vi "ejer9.vi"() -> ()   [LabVIEW 2014]
panel:
  out "Circuito resonante":bool
  in  "VRMS":dbl
  in  "Fase de V":dbl
  in  "Frec del V":dbl
  in  "Resistencia.":dbl
  in  "Capacitancia":dbl
  in  "Inductancia":dbl
  out "Voltaje Fuente":dynamicdata(graph) caption="Sine"
  out "Corriente Circuito":dynamicdata(graph) caption="Sine"
  out "Voltaje  Inductor":dynamicdata(graph) caption="Sine"
  out "Voltaje Capacitor":dynamicdata(graph) caption="Sine"
  out "Voltaje  Resistencia":dynamicdata(graph) caption="Sine"
  out "Impedancia":cdb
  out "Frec de Resonancia.":dbl
  out "IRMS":dbl
  out "Fase de I":dbl
  out "V Inductor":cdb
  out "V Capacitor":cdb
  out "V Resistencia":cdb
  in  "stop":bool
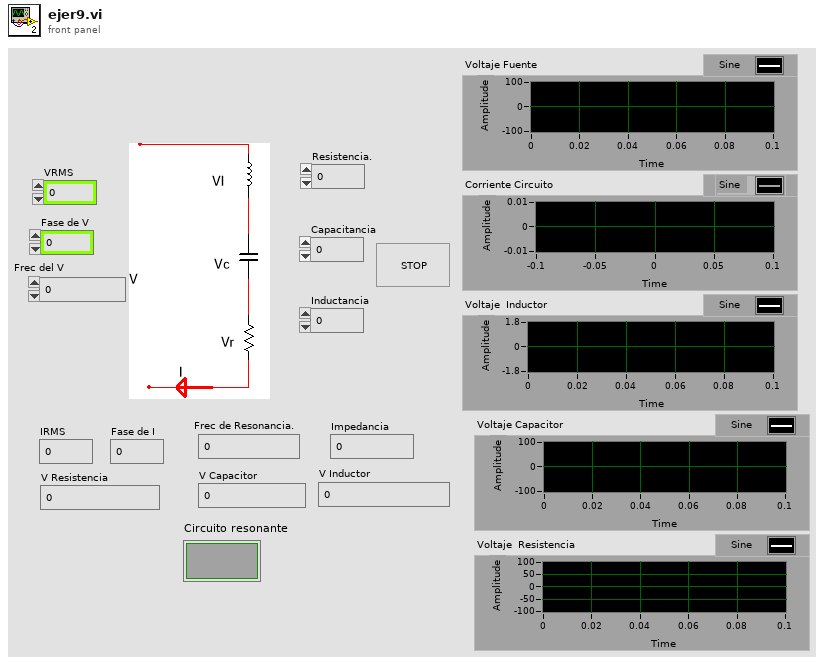
[diagram p1: front panel]
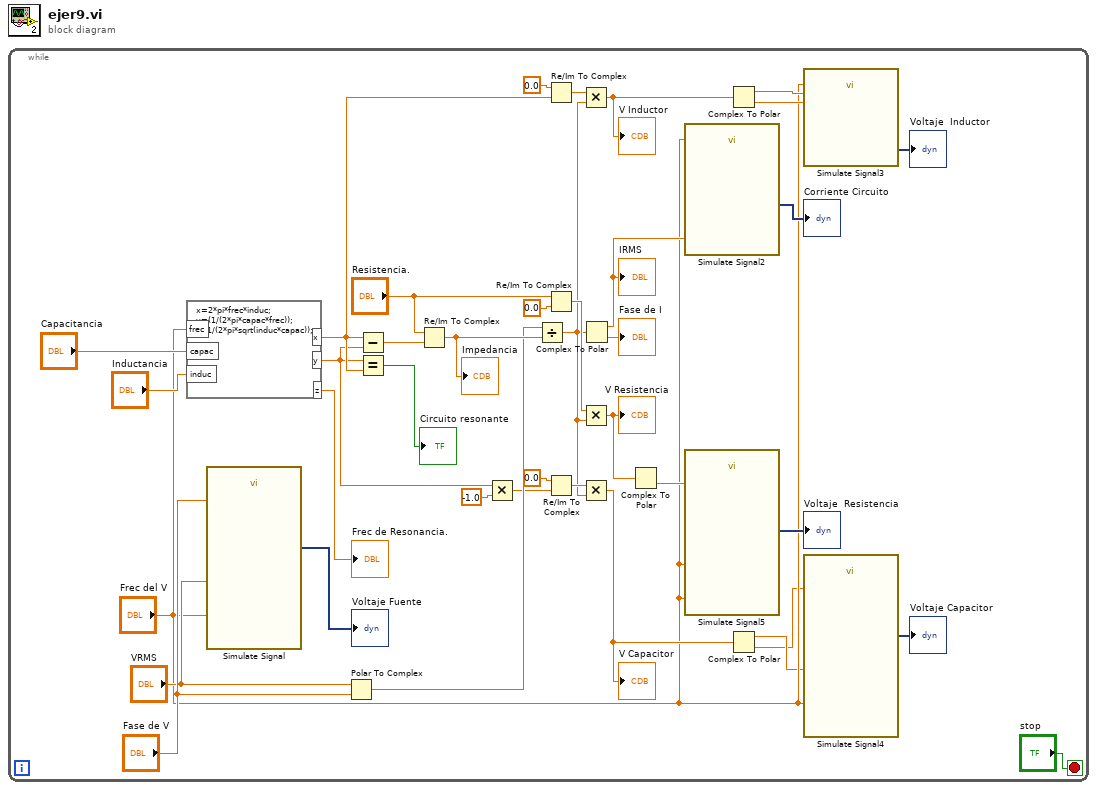
[diagram p0: block diagram]
diagram:
  n1 = while {
    stop <- "stop" stop-if-true
    n2 = formula code="x=2*pi*frec*induc;\ny=(1/(2*pi*capac*frec));\nz=1/(2*pi*sqrt(induc*capac));"("frec"="Frec del V", "induc"="Inductancia", "capac"="Capacitancia") -> ("x"=w10:dbl, "y"=w8:dbl, "z"=→"Frec de Resonancia.":dbl)
    n3 = call "Simulate Signal"("Frequency"="Frec del V", "Amplitude"="VRMS", "Phase"="Fase de V") -> ("Sine"=→"Voltaje Fuente":dynamicdata)  [unwired: 11 in, 1 out]
    n4 = Polar To Complex(1:"Fase de V", 2:"VRMS") -> (0:w34:cdb)
    n5 = Subtract(x=w10, y=w8) -> (x-y=w37:dbl)
    n6 = Equal?(x=w8, y=w10) -> (x = y?=→"Circuito resonante":bool)
    n7 = Re/Im To Complex(1:w37, 2:"Resistencia.") -> (0:w35:cdb)
    "Impedancia" <- w35
    n8 = Multiply(x=w8, y=-1.0) -> (x*y=w30:dbl)
    n9 = Divide(x=w34, y=w35) -> (x/y=w1:cdb)
    n10 = Re/Im To Complex(1:w10, 2:0.0 ("x")) -> (0:w29:cdb)
    n11 = Re/Im To Complex(1:0.0 ("y"), 2:"Resistencia.") -> (0:w25:cdb)
    n12 = Re/Im To Complex(1:w30, 2:0.0 ("x")) -> (0:w28:cdb)
    n13 = Multiply(x=w29, y=w1) -> (x*y=w20:cdb)
    "V Inductor" <- w20
    n14 = Multiply(x=w25, y=w1) -> (x*y=w6:cdb)
    "V Resistencia" <- w6
    n15 = Multiply(x=w28, y=w1) -> (x*y=w17:cdb)
    "V Capacitor" <- w17
    n16 = Complex To Polar(r * e^(i*theta)=w1) -> (r=w21:dbl, theta=→"Fase de I":dbl)
    "IRMS" <- w21
    n17 = Complex To Polar(r * e^(i*theta)=w6) -> (theta=w16:dbl)  [unwired: 1 out]
    n18 = call "Simulate Signal2"("Frequency"="Frec del V", "Amplitude"=w21) -> ("Sine"=→"Corriente Circuito":dynamicdata)  [unwired: 12 in, 1 out]
    n19 = call "Simulate Signal5"("Frequency"="Frec del V", "Amplitude"="Frec del V", "Phase"=w16) -> ("Sine"=→"Voltaje  Resistencia":dynamicdata)  [unwired: 11 in, 1 out]
    n20 = Complex To Polar(r * e^(i*theta)=w20) -> (r=w19:dbl, theta=w18:dbl)
    n21 = Complex To Polar(r * e^(i*theta)=w17) -> (r=w3:dbl, theta=w2:dbl)
    n22 = call "Simulate Signal3"("Frequency"="Frec del V", "Amplitude"=w19, "Phase"=w18) -> ("Sine"=→"Voltaje  Inductor":dynamicdata)  [unwired: 11 in, 1 out]
    n23 = call "Simulate Signal4"("Frequency"="Frec del V", "Amplitude"=w3, "Phase"=w2) -> ("Sine"=→"Voltaje Capacitor":dynamicdata)  [unwired: 11 in, 1 out]
  }
